vi "Response Error and Data.vi"(8 "error in (no error)":errorcluster, 9 "Data In":variant, 10 "Message":string, 11 "Name":string) -> (0 "error out":errorcluster, 1 "Last Data":variant, 2 "last notification":errorcluster)   [LabVIEW 2019, in "Data and Error Notifier.lvlib"]
uses:
  Data and Error Notifier.lvlib
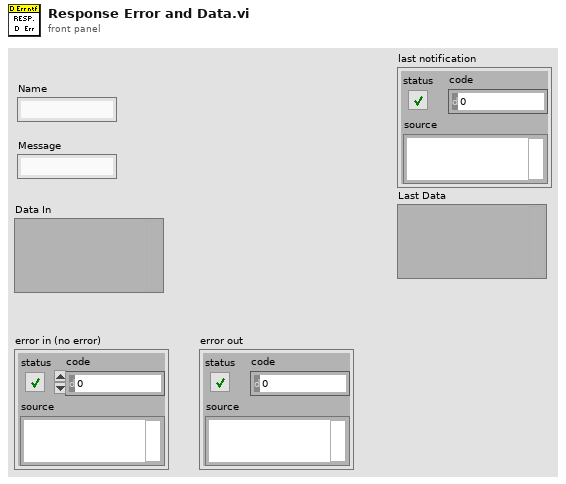
[diagram p1: front panel]
types:
  T1 = typedef "Data and Error Notifier.lvlib/Data Error cluster.ctl" = cluster{"Data":variant, "Error":errorcluster}
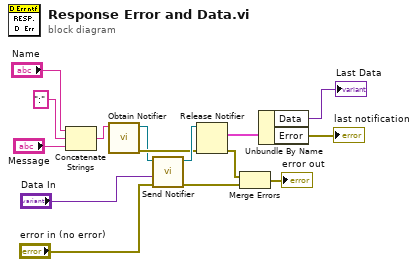
[diagram p0: block diagram]
diagram:
  n1 = Concatenate Strings("Name", ":" ("string"), "Message") -> (w5:string)
  n2 = call "Obtain Notifier.vi"("Name"=w5) -> ("Error Out"=w11:errorcluster, "notifier out"=w9:refnum<notifier>)  [unwired: 9 in]
  n3 = call "Send Notifier.vi"("Error In"="error in (no error)", "Data In"="Data In", "notifier in"=w9) -> ("Error Out"=w15:errorcluster, "notifier out"=w12:refnum<notifier>)  [unwired: 7 in]
  n4 = Release Notifier(notifier=w12, error in (no error)=w11) -> (last notification=w4:T1, error out=w14:errorcluster)  [unwired: 1 in, 1 out]
  n5 = Merge Errors(w14, w15) -> (→"error out":errorcluster)
  n6 = Unbundle By Name(w4) -> ("Data"=→"Last Data":variant, "Error"=→"last notification":errorcluster)
